vi "Check eeprom.vi"() -> ()   [LabVIEW 2015]
panel:
  in  "milliseconds to wait":u32
  in  "Stop Button":bool
  out "XY Graph":cluster{dbl[], i32[]}[](graph)
  out "number 2":i32
  out "number":i32
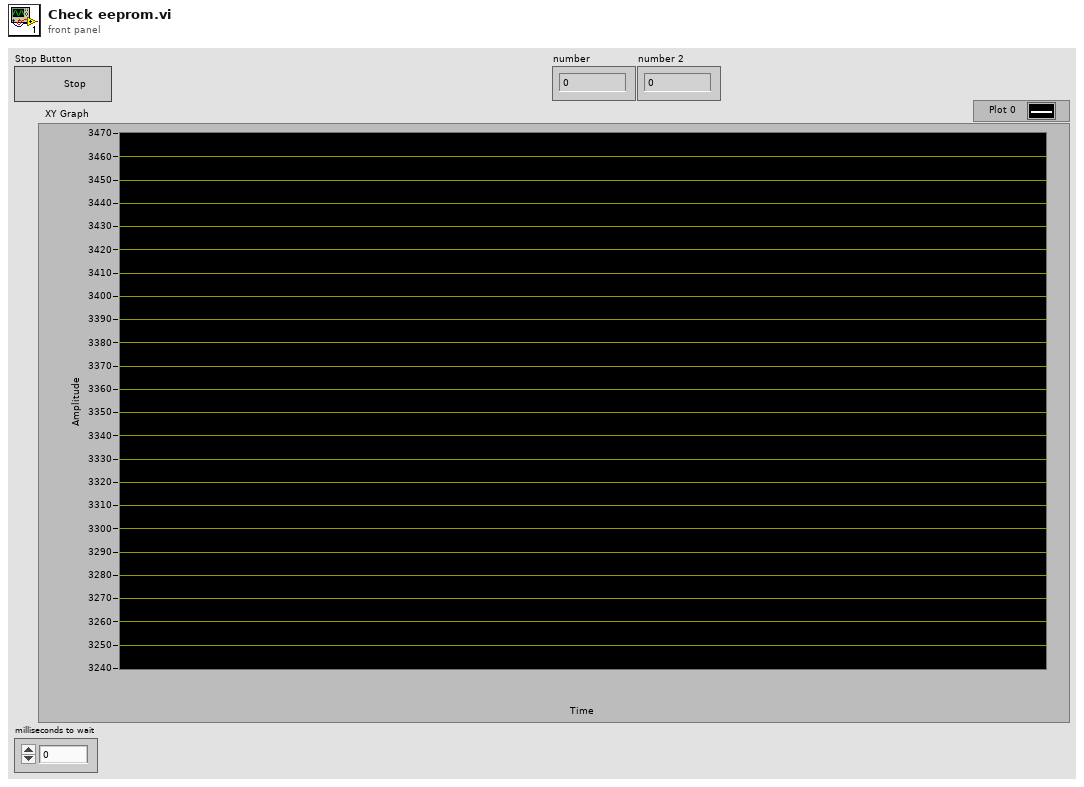
[diagram p1: front panel]
types:
  T1 = enum16{"Read", "Write", "ReadWrite", "BufferedRead", "BufferedReadWrite"}
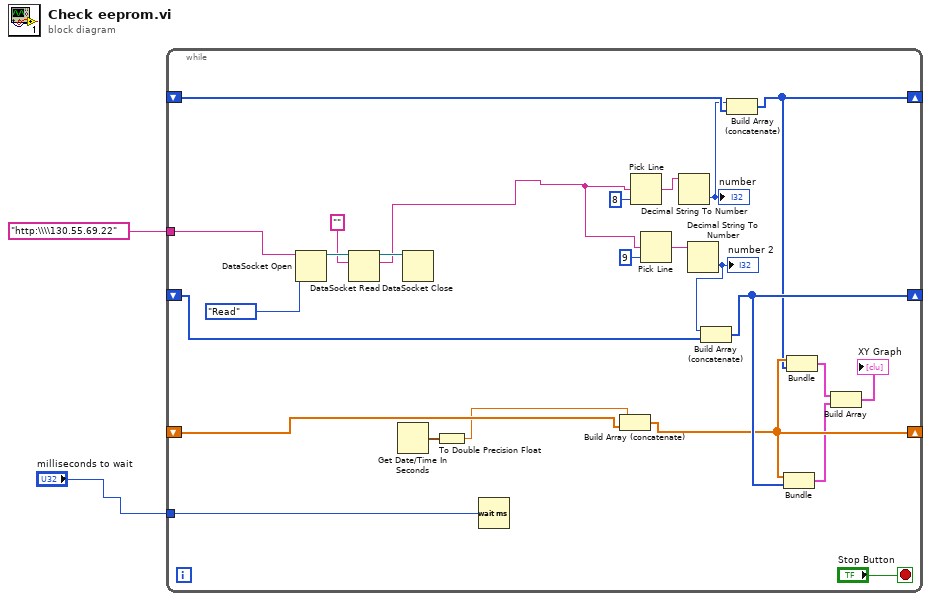
[diagram p0: block diagram]
diagram:
  n1 = while {
    tunnel: "http:\\\\130.55.69.22" ("URL") -> [w27]
    shift-right: [w8] -> _
    shift-left: _ -> [w16]
    shift-right: [w10] -> _
    shift-left: _ -> [w13]
    shift-right: [w9] -> _
    shift-left: _ -> [w12]
    tunnel: "milliseconds to wait" -> [w3]
    stop <- "Stop Button" stop-if-true
    n2 = DataSocket Open(10:T1."Read" ("mode"), 11:w27) -> (3:w26:refnum<k13>)  [unwired: 2 in, 1 out]
    n3 = DataSocket Read(10:"" ("URL"), 11:w26) -> (2:w20:string, 3:w25:refnum<k13>)  [unwired: 3 in, 5 out]
    n4 = Get Date/Time In Seconds() -> (seconds since 1Jan1904=w17:timestamp)
    n5 = DataSocket Close(11:w25) -> ()  [unwired: 2 in, 2 out]
    n6 = To Double Precision Float(number=w17) -> (double precision float=w11:dbl)
    n7 = Wait (ms)(milliseconds to wait=w3) -> ()  [unwired: 1 out]
    n8 = Build Array (concatenate)(w11, w12) -> (w9:dbl[])
    n9 = Pick Line(multi-line string=w20, line index=8) -> (output string=w19:string)  [unwired: 1 in]
    n10 = Pick Line(multi-line string=w20, line index=9) -> (output string=w18:string)  [unwired: 1 in]
    n11 = Decimal String To Number(string=w19) -> (number=w15:i32)  [unwired: 2 in, 1 out]
    "number" <- w15
    n12 = Decimal String To Number(string=w18) -> (number=w14:i32)  [unwired: 2 in, 1 out]
    "number 2" <- w14
    n13 = Build Array (concatenate)(w14, w13) -> (w10:i32[])
    n14 = Build Array (concatenate)(w15, w16) -> (w8:i32[])
    n15 = Bundle(w9, w10) -> (w6:cluster{dbl[], i32[]})  [unwired: 1 in]
    n16 = Bundle(w9, w8) -> (w7:cluster{dbl[], i32[]})  [unwired: 1 in]
    n17 = Build Array(w7, w6) -> (→"XY Graph":cluster{dbl[], i32[]}[])
  }
